vi "niDTS BT INSTR TX Configure Hardware Parameters.vi"(8 "error in (no error)":errorcluster, 10 "MaxInputPower":dbl, 11 "niDTS BT INSTR TX in":refnum<class "niDTS BT INSTR TX.lvclass">) -> (0 "error out":errorcluster, 3 "niDTS BT INSTR TX out":refnum<class "niDTS BT INSTR TX.lvclass">)   [LabVIEW 2015, in "niDTS BT.lvlib" / "niDTS BT INSTR TX.lvclass"]
uses:
  niDTS BT INSTR TX.lvclass
  niDTS BT INSTR TX.lvclass/niDTS BT INSTR TX.ctl
  RiviInstDriver/niRfsaBT/Objects/niRfsaBt.lvclass
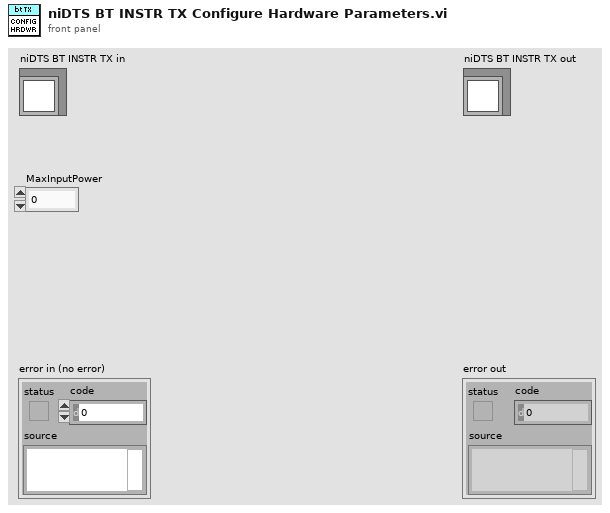
[diagram p1: front panel]
types:
  T1 = typedef "niRfsaBT.lvclass/niRfsaBT INC Handle.ctl" = refnum<data-value>
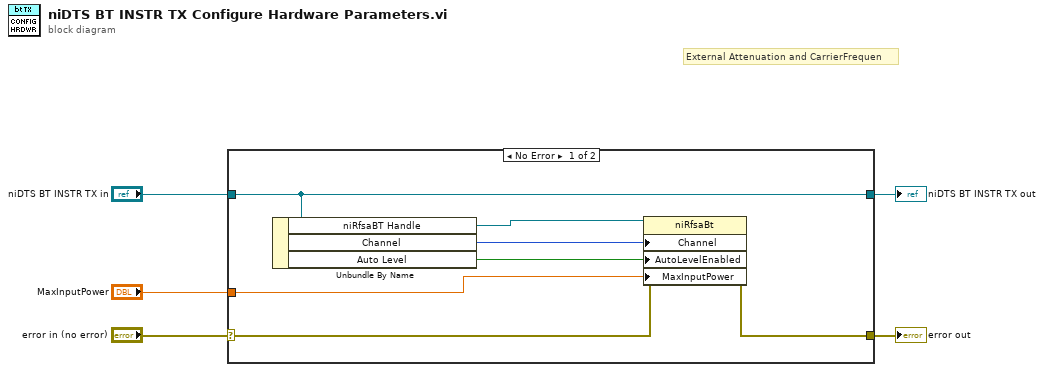
[diagram p0: block diagram]
diagram:
  # "External Attenuation and CarrierFrequen"
  n1 = case shown="No Error" "error in (no error)" {
    selector: "error in (no error)" -> [w11 w14]
    tunnel: [w10 w14] -> w4
    tunnel: [w12 w13] -> w2
    tunnel: "niDTS BT INSTR TX in" -> [w12 w13]
    tunnel: "MaxInputPower" -> [w6 _]
    frame No Error {
      n2 = Unbundle By Name(w12) -> ("niRfsaBT Handle"=w9:T1, "Channel"=w8:i32, "Auto Level"=w7:bool)
      n3 = property class="niRfsaBt"(reference=w9, error in=w11, "Channel"=w8, "AutoLevelEnabled"=w7, "MaxInputPower"=w6) -> (error out=w10:errorcluster)  [unwired: 1 out]
    }
    frame Error {
    }
  }
  "error out" <- w4
  "niDTS BT INSTR TX out" <- w2
